vi "Pre-Build Custom Action.vi"(10 "Variant":variant) -> (0 "error out":errorcluster)   [LabVIEW 2017]
uses:
  <vilib>/addons/_JKI Toolkits/Caraya/run-tests/Run Test (Scalar Path).vi
  <vilib>/addons/_JKI Toolkits/Caraya/Caraya.lvlib
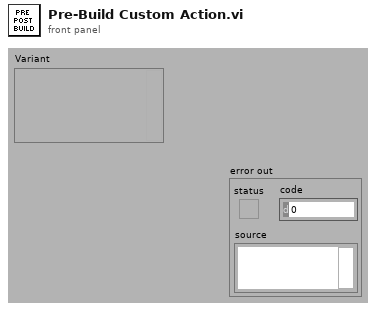
[diagram p1: front panel]
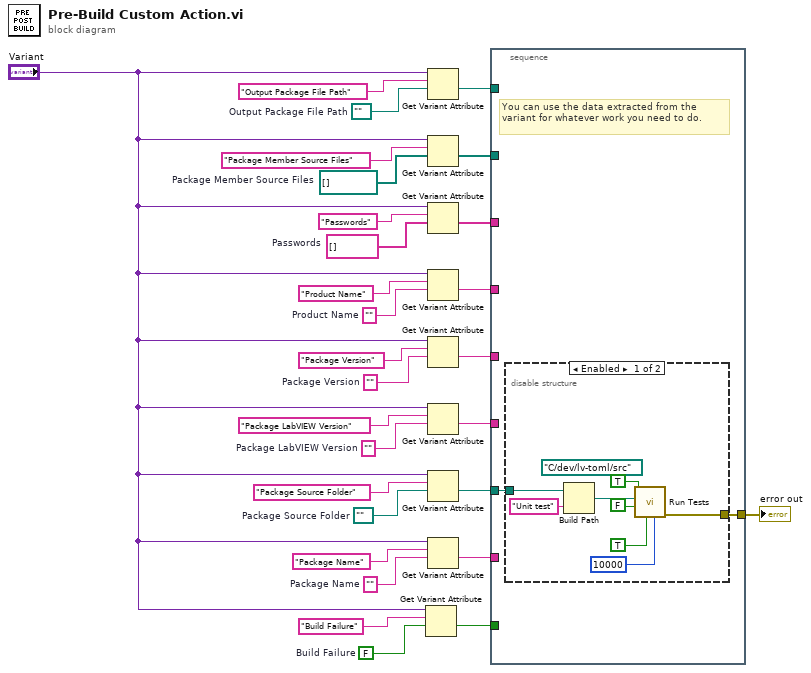
[diagram p0: block diagram]
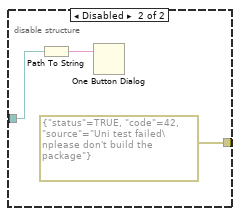
[diagram p2: hidden frame]
diagram:
  w5 = FALSE  # Build Failure
  w14 = path ""  # Package Source Folder
  w15 = ""  # Package Name
  w18 = ""  # Package LabVIEW Version
  w20 = ""  # Package Version
  w22 = ""  # Product Name
  w24 = string[] []  # Passwords
  w26 = path[] []  # Package Member Source Files
  w28 = path ""  # Output Package File Path
  n1 = Get Variant Attribute(Variant="Variant", name="Build Failure", default value (empty Variant)=w5) -> (value=w3:bool)  [unwired: 1 in, 3 out]
  n2 = Get Variant Attribute(Variant="Variant", name="Output Package File Path", default value (empty Variant)=w28) -> (value=w13:path)  [unwired: 1 in, 3 out]
  n3 = Get Variant Attribute(Variant="Variant", name="Package Member Source Files", default value (empty Variant)=w26) -> (value=w12:path[])  [unwired: 1 in, 3 out]
  n4 = Get Variant Attribute(Variant="Variant", name="Passwords", default value (empty Variant)=w24) -> (value=w11:string[])  [unwired: 1 in, 3 out]
  n5 = Get Variant Attribute(Variant="Variant", name="Product Name", default value (empty Variant)=w22) -> (value=w10:string)  [unwired: 1 in, 3 out]
  n6 = Get Variant Attribute(Variant="Variant", name="Package Version", default value (empty Variant)=w20) -> (value=w9:string)  [unwired: 1 in, 3 out]
  n7 = Get Variant Attribute(Variant="Variant", name="Package LabVIEW Version", default value (empty Variant)=w18) -> (value=w8:string)  [unwired: 1 in, 3 out]
  n8 = Get Variant Attribute(Variant="Variant", name="Package Source Folder", default value (empty Variant)=w14) -> (value=w1:path)  [unwired: 1 in, 3 out]
  n9 = Get Variant Attribute(Variant="Variant", name="Package Name", default value (empty Variant)=w15) -> (value=w7:string)  [unwired: 1 in, 3 out]
  n10 = stacked-sequence {
    tunnel: w13 -> [_]
    tunnel: w12 -> [_]
    tunnel: w11 -> [_]
    tunnel: w10 -> [_]
    tunnel: w9 -> [_]
    tunnel: w8 -> [_]
    tunnel: w1 -> [w31]
    tunnel: w7 -> [_]
    tunnel: w3 -> [_]
    tunnel: [w30] -> w2
    frame #0 {
      # "You can use the data extracted from the variant for whatever work you need to do."
      n11 = disable-structure shown="Enabled" {
        disable-tunnel: w31 -> [w39 w41]
        disable-tunnel: [w32 errorcluster {"status"=TRUE, "code"=42, "source"="Uni test failed\nplease don't build the package"} ("error out")] -> w30
        frame Enabled {
          (unwired) path "C:/dev/lv-toml/src"
          n12 = Build Path(base path=w39, name or relative path="Unit test") -> (appended path=w35:path)
          n13 = call-poly <vilib>:"Run Tests.vi"("timeout (2000 ms)"=10000, "Verbose"=TRUE, "Inspect Recursively (T)"=FALSE ("Interactive (T)"), "Test Path"=w35, "Interactive (T)"=TRUE) -> ("error out"=w32:errorcluster)  [unwired: 6 in]
        }
        frame Disabled {
          n14 = Path To String(path=w41) -> (string=w40:string)
          n15 = One Button Dialog(message=w40) -> ()  [unwired: 1 in, 1 out]
        }
      }
    }
  }
  "error out" <- w2
